vi "Update Channels on Change.vi"(10 "new channel table":T1[](array[typedef]) {"input terminal configuration" items=["default"=-1, "RSE"=10083, "NRSE"=10078, "Differential"=10106, "Pseudodifferential"=12529]; "Channel Type" items=["Voltage (V)"=0, "Charge (C)"=9, "-"=99, "SPL (Pa)"=3, "Force (lbf)"=6, "Force (N)"=1, "Acceleration (g) - IEPE"=2, "Acceleration (g) - Charge"=12, "Acceleration (g) - 4 wire DC Voltage"=22, "Velocity (in/s)"=7, "Velocity (mm/s)"=8, "Prox Probe (mil)"=4, "Prox Probe (mm)"=5]}, 11 "old channel table":T1[](array[typedef]) {"input terminal configuration" items=["default"=-1, "RSE"=10083, "NRSE"=10078, "Differential"=10106, "Pseudodifferential"=12529]; "Channel Type" items=["Voltage (V)"=0, "Charge (C)"=9, "-"=99, "SPL (Pa)"=3, "Force (lbf)"=6, "Force (N)"=1, "Acceleration (g) - IEPE"=2, "Acceleration (g) - Charge"=12, "Acceleration (g) - 4 wire DC Voltage"=22, "Velocity (in/s)"=7, "Velocity (mm/s)"=8, "Prox Probe (mil)"=4, "Prox Probe (mm)"=5]}) -> (3 "updated channel table":T1[](array[typedef]) {"input terminal configuration" items=["default"=-1, "RSE"=10083, "NRSE"=10078, "Differential"=10106, "Pseudodifferential"=12529]; "Channel Type" items=["Voltage (V)"=0, "Charge (C)"=9, "-"=99, "SPL (Pa)"=3, "Force (lbf)"=6, "Force (N)"=1, "Acceleration (g) - IEPE"=2, "Acceleration (g) - Charge"=12, "Acceleration (g) - 4 wire DC Voltage"=22, "Velocity (in/s)"=7, "Velocity (mm/s)"=8, "Prox Probe (mil)"=4, "Prox Probe (mm)"=5]})   [LabVIEW 2024, in "Dynamic Signal Acquisition (Interactive) UI.lvlib"]
uses:
  SFPDAQmx Channel Info.ctl
  <vilib>/addons/Sound and Vibration/svt_DAQmx/Configuration XControl/Controls/svx_DAQ_Excitation.ctl
  <vilib>/addons/Sound and Vibration/svt_DAQmx/Configuration XControl/Controls/svx_DAQ_Coupling.ctl
  <vilib>/addons/Sound and Vibration/svt_DAQmx/Configuration XControl/Controls/svx_DAQ_ChannelType.ctl
  <vilib>/DAQmx/create/channels.llb/DAQmx Create Channel (TEDS-AI-Sound Pressure-Microphone).vi
  <vilib>/DAQmx/create/channels.llb/DAQmx Create Channel (TEDS-AI-Force-IEPE Sensor).vi
  <vilib>/DAQmx/create/channels.llb/DAQmx Create Channel (TEDS-AI-Acceleration-Accelerometer).vi
  Dynamic Signal Acquisition (Interactive) UI.lvlib
  <vilib>/addons/Sound and Vibration/svt_DAQmx/Configuration XControl/SVX NI-DAQmx AI Configuration XControl.xctl
  <resource>/objmgr/daqmx.rc
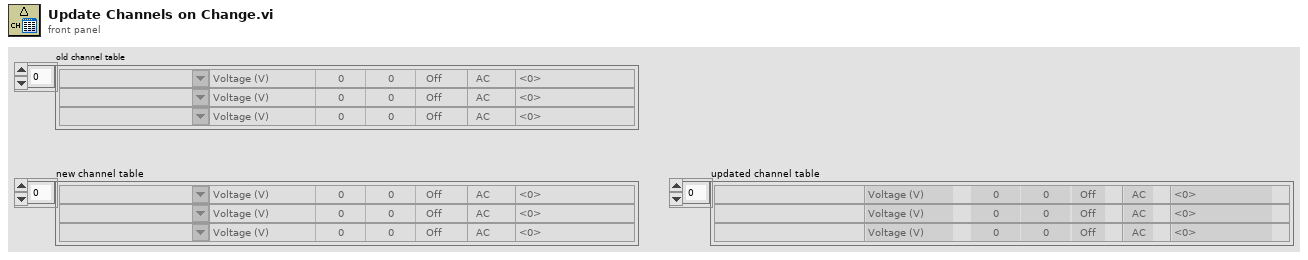
[diagram p1: front panel]
types:
  T1 = typedef "Dynamic Signal Acquisition (Interactive) UI.lvlib/SFPDAQmx Channel Info.ctl" = cluster{"DAQmx Channel":tag, "Channel Type":u16, "Max":dbl, "Sensitivity":dbl, "Coupling":enum16{"AC", "DC"}, "input terminal configuration":i32, "excitation":enum16{"Off", "Min", "Max"}}
  T2 = typedef "svx_DAQ_Excitation.ctl" = enum16{"Off", "Min", "Max"}
  T3 = typedef "SVX NI-DAQmx AI Configuration XControl.xctl/svx_DAQ_Coupling.ctl" = enum16{"AC", "DC"}
  T4 = typedef "SVX NI-DAQmx AI Configuration XControl.xctl/svx_DAQ_ChannelType.ctl" = u16
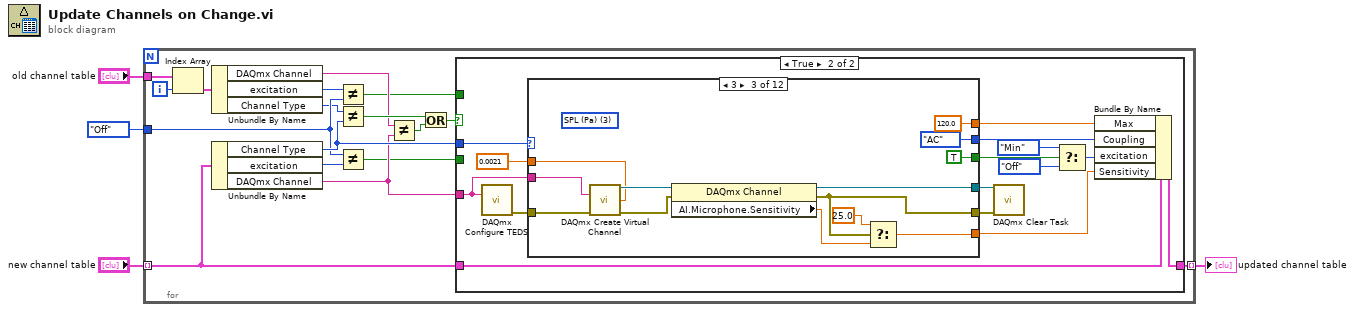
[diagram p0: block diagram]
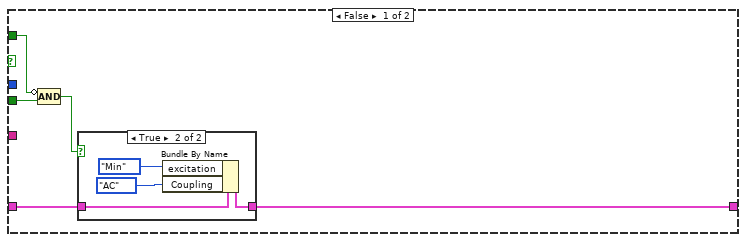
[diagram p2: hidden frame]
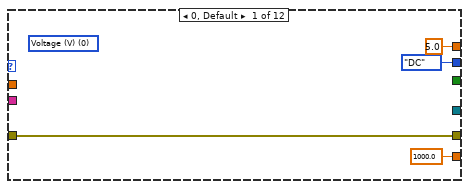
[diagram p4: hidden frame]
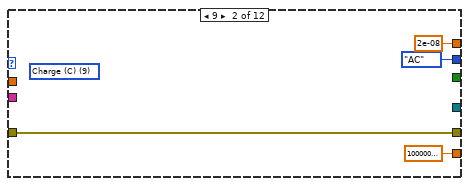
[diagram p5: hidden frame]
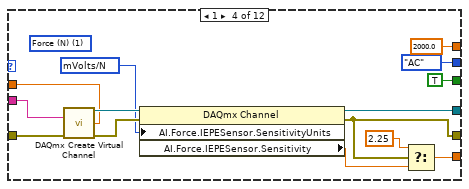
[diagram p6: hidden frame]
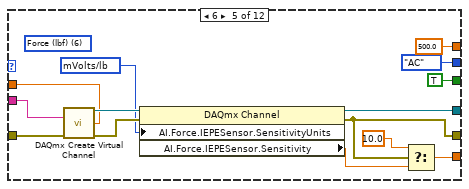
[diagram p7: hidden frame]
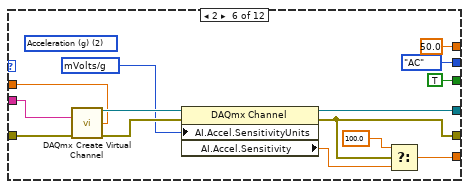
[diagram p8: hidden frame]
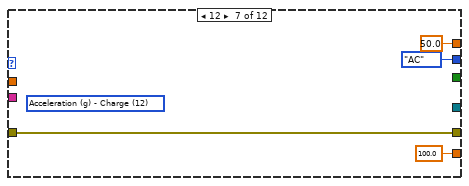
[diagram p9: hidden frame]
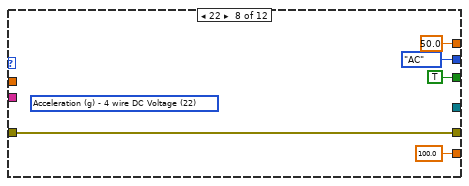
[diagram p10: hidden frame]
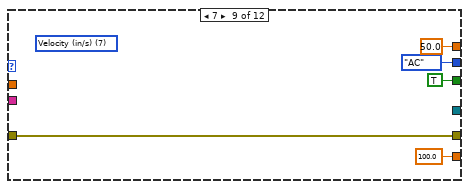
[diagram p11: hidden frame]
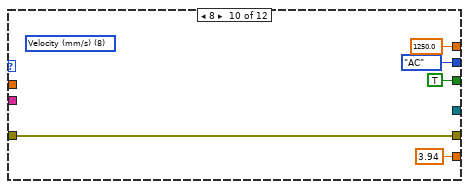
[diagram p12: hidden frame]
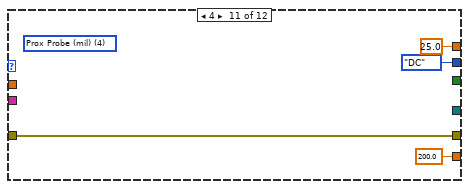
[diagram p13: hidden frame]
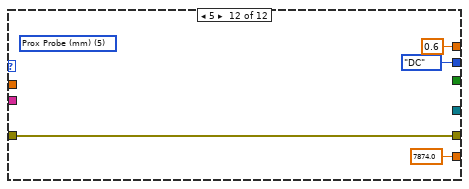
[diagram p14: hidden frame]
diagram:
  n1 = for {
    tunnel: "new channel table" -> [w21] mode=indexing
    tunnel: [w17] -> w2 mode=indexing
    tunnel: "old channel table" -> [w20]
    tunnel: svx_DAQ_Excitation."Off" ("y") -> [w13]
    i -> [w19]
    n2 = Index Array(array=w20, index=w19) -> (element=w18:T1)
    n3 = Unbundle By Name(w18) -> ("DAQmx Channel"=w10:tag, "excitation"=w14:enum16{"Off", "Min", "Max"}, "Channel Type"=w12:u16)
    n4 = Unbundle By Name(w21) -> ("Channel Type"=w16:u16, "excitation"=w15:enum16{"Off", "Min", "Max"}, "DAQmx Channel"=w9:tag)
    n5 = Not Equal?(x=w14, y=w13) -> (x != y?=w5:bool)
    n6 = Not Equal?(x=w12, y=w16) -> (x != y?=w11:bool)
    n7 = Not Equal?(x=w13, y=w15) -> (x != y?=w6:bool)
    n8 = Not Equal?(x=w10, y=w9) -> (x != y?=w8:bool)
    n9 = Or(x=w11, y=w8) -> (x .or. y?=w7:bool)
    n10 = case shown="True" w7 {
      tunnel: w21 -> [w23 w46]
      tunnel: [w22 w45] -> w17
      tunnel: w16 -> [_ w44]
      tunnel: w5 -> [w26 _]
      tunnel: w6 -> [w25 _]
      tunnel: w9 -> [_ w37]
      frame False {
        n11 = Compound Arithmetic op=AND(invert w26, w25) -> (w24:bool)
        n12 = case shown="True" w24 {
          tunnel: w23 -> [w27 w31]
          tunnel: [w27 w30] -> w22
          frame False {
          }
          frame True {
            n13 = Bundle By Name(cluster=w31, "excitation"=svx_DAQ_Excitation."Min", "Coupling"=svx_DAQ_Coupling."AC") -> (w30:T1)
          }
        }
      }
      frame True {
        n14 = call <vilib>:"DAQmx Configure TEDS.vi"("physical channel"=w37) -> ("error out"=w35:errorcluster)  [unwired: 14 in]
        n15 = case shown="3" w44 {
          tunnel: [5.0 ("Max") 2e-08 ("Max") 120.0 ("Max") 2000.0 ("Max") 500.0 ("Max") 50.0 ("Max") 50.0 ("Max") 50.0 ("Max") 50.0 ("Max") 1250.0 ("Max") 25.0 ("Max") 0.6 ("Max")] -> w43
          tunnel: [1000.0 ("Sensitivity") 1000000000000.0 ("Sensitivity") w56 w70 w83 w97 100.0 ("Sensitivity") 100.0 ("Sensitivity") 100.0 ("Sensitivity") 3.94 ("Sensitivity") 200.0 ("Sensitivity") 7874.0 ("Sensitivity")] -> w33
          tunnel: [svx_DAQ_Coupling."DC" ("Coupling") svx_DAQ_Coupling."AC" ("Coupling") svx_DAQ_Coupling."AC" ("Coupling") svx_DAQ_Coupling."AC" ("Coupling") svx_DAQ_Coupling."AC" ("Coupling") svx_DAQ_Coupling."AC" ("Coupling") svx_DAQ_Coupling."AC" ("Coupling") svx_DAQ_Coupling."AC" ("Coupling") svx_DAQ_Coupling."AC" ("Coupling") svx_DAQ_Coupling."AC" ("Coupling") svx_DAQ_Coupling."DC" ("Coupling") svx_DAQ_Coupling."DC" ("Coupling")] -> w42
          tunnel: [_ _ TRUE ("IEPE") TRUE ("IEPE") TRUE ("IEPE") TRUE ("IEPE") _ TRUE ("IEPE") TRUE ("IEPE") TRUE ("IEPE") _ _] -> w39
          tunnel: w37 -> [_ _ w64 w72 w87 w99 _ _ _ _ _ _]
          tunnel: [_ _ w62 w69 w86 w101 _ _ _ _ _ _] -> w36
          tunnel: w35 -> [w47 w51 w61 w73 w88 w102 w110 w114 w119 w124 w129 w133]
          tunnel: [w47 w51 w59 w71 w85 w100 w110 w114 w119 w124 w129 w133] -> w34
          tunnel: 0.0021 ("current excitation value") -> [_ _ w55 w68 w82 w96 _ _ _ _ _ _]
          frame 0, Default {
            (unwired) T4 0 items=["Voltage (V)"=0, "SPL (Pa)"=3, "Force (lbf)"=6, "Force (N)"=1, "Acceleration (g)"=2, "Velocity (in/s)"=7, "Velocity (mm/s)"=8, "Prox Probe (mil)"=4, "Prox Probe (mm)"=5] ("Channel Type")
          }
          frame 9 {
            (unwired) T4 9 items=["Voltage (V)"=0, "Charge (C)"=9, "-"=99, "SPL (Pa)"=3, "Force (lbf)"=6, "Force (N)"=1, "Acceleration (g) - IEPE"=2, "Acceleration (g) - Charge"=12, "Acceleration (g) - 4 wire DC Voltage"=22, "Velocity (in/s)"=7, "Velocity (mm/s)"=8, "Prox Probe (mil)"=4, "Prox Probe (mm)"=5] ("Channel Type")
          }
          frame 3 {
            (unwired) T4 3 items=["Voltage (V)"=0, "SPL (Pa)"=3, "Force (lbf)"=6, "Force (N)"=1, "Acceleration (g)"=2, "Velocity (in/s)"=7, "Velocity (mm/s)"=8, "Prox Probe (mil)"=4, "Prox Probe (mm)"=5] ("Channel Type")
            n16 = call-poly <vilib>:"DAQmx Create Virtual Channel.vi"("physical channels"=w64, "current excitation value"=w55, "error in"=w61) -> ("task out"=w63:refnum<k21>, "error out"=w60:errorcluster)  [unwired: 11 in]
            n17 = property class="DAQmx Channel"(reference=w63, error in=w60) -> (reference out=w62:refnum<k21>, error out=w59:errorcluster, "AI.Microphone.Sensitivity"=w58:dbl)
            n18 = Select(t=25.0 ("Sensitivity"), s=w59, f=w58) -> (s? t:f=w56:dbl)
          }
          frame 1 {
            w74 = 15891 items=["mVolts/N"=15891, "mVolts/lb"=15892] ("AI.Force.IEPESensor.SensitivityUnits")
            (unwired) T4 1 items=["Voltage (V)"=0, "SPL (Pa)"=3, "Force (lbf)"=6, "Force (N)"=1, "Acceleration (g)"=2, "Velocity (in/s)"=7, "Velocity (mm/s)"=8, "Prox Probe (mil)"=4, "Prox Probe (mm)"=5] ("Channel Type")
            n19 = call-poly <vilib>:"DAQmx Create Virtual Channel.vi"("physical channels"=w72, "current excitation value"=w68, "error in"=w73) -> ("task out"=w78:refnum<k21>, "error out"=w77:errorcluster)  [unwired: 11 in]
            n20 = property class="DAQmx Channel"(reference=w78, error in=w77, "AI.Force.IEPESensor.SensitivityUnits"=w74) -> (reference out=w69:refnum<k21>, error out=w71:errorcluster, "AI.Force.IEPESensor.Sensitivity"=w76:dbl)
            n21 = Select(t=2.25 ("Sensitivity"), s=w71, f=w76) -> (s? t:f=w70:dbl)
          }
          frame 6 {
            w84 = 15892 items=["mVolts/N"=15891, "mVolts/lb"=15892] ("AI.Force.IEPESensor.SensitivityUnits")
            (unwired) T4 6 items=["Voltage (V)"=0, "SPL (Pa)"=3, "Force (lbf)"=6, "Force (N)"=1, "Acceleration (g)"=2, "Velocity (in/s)"=7, "Velocity (mm/s)"=8, "Prox Probe (mil)"=4, "Prox Probe (mm)"=5] ("Channel Type")
            n22 = call-poly <vilib>:"DAQmx Create Virtual Channel.vi"("physical channels"=w87, "current excitation value"=w82, "error in"=w88) -> ("task out"=w92:refnum<k21>, "error out"=w91:errorcluster)  [unwired: 11 in]
            n23 = property class="DAQmx Channel"(reference=w92, error in=w91, "AI.Force.IEPESensor.SensitivityUnits"=w84) -> (reference out=w86:refnum<k21>, error out=w85:errorcluster, "AI.Force.IEPESensor.Sensitivity"=w90:dbl)
            n24 = Select(t=10.0 ("Sensitivity"), s=w85, f=w90) -> (s? t:f=w83:dbl)
          }
          frame 2 {
            w103 = 12509 items=["mVolts/g"=12509, "Volts/g"=12510] ("AI.Accel.SensitivityUnits")
            (unwired) T4 2 items=["Voltage (V)"=0, "SPL (Pa)"=3, "Force (lbf)"=6, "Force (N)"=1, "Acceleration (g)"=2, "Velocity (in/s)"=7, "Velocity (mm/s)"=8, "Prox Probe (mil)"=4, "Prox Probe (mm)"=5] ("Channel Type")
            n25 = call-poly <vilib>:"DAQmx Create Virtual Channel.vi"("physical channels"=w99, "current excitation value"=w96, "error in"=w102) -> ("task out"=w106:refnum<k21>, "error out"=w105:errorcluster)  [unwired: 11 in]
            n26 = property class="DAQmx Channel"(reference=w106, error in=w105, "AI.Accel.SensitivityUnits"=w103) -> (reference out=w101:refnum<k21>, error out=w100:errorcluster, "AI.Accel.Sensitivity"=w104:dbl)
            n27 = Select(t=100.0 ("Sensitivity"), s=w100, f=w104) -> (s? t:f=w97:dbl)
          }
          frame 12 {
            (unwired) T4 12 items=["Voltage (V)"=0, "Charge (C)"=9, "-"=99, "SPL (Pa)"=3, "Force (lbf)"=6, "Force (N)"=1, "Acceleration (g) - IEPE"=2, "Acceleration (g) - Charge"=12, "Acceleration (g) - 4 wire DC Voltage"=22, "Velocity (in/s)"=7, "Velocity (mm/s)"=8, "Prox Probe (mil)"=4, "Prox Probe (mm)"=5] ("Channel Type")
          }
          frame 22 {
            (unwired) T4 22 items=["Voltage (V)"=0, "Charge (C)"=9, "-"=99, "SPL (Pa)"=3, "Force (lbf)"=6, "Force (N)"=1, "Acceleration (g) - IEPE"=2, "Acceleration (g) - Charge"=12, "Acceleration (g) - 4 wire DC Voltage"=22, "Velocity (in/s)"=7, "Velocity (mm/s)"=8, "Prox Probe (mil)"=4, "Prox Probe (mm)"=5] ("Channel Type")
          }
          frame 7 {
            (unwired) T4 7 items=["Voltage (V)"=0, "SPL (Pa)"=3, "Force (lbf)"=6, "Force (N)"=1, "Acceleration (g)"=2, "Velocity (in/s)"=7, "Velocity (mm/s)"=8, "Prox Probe (mil)"=4, "Prox Probe (mm)"=5] ("Channel Type")
          }
          frame 8 {
            (unwired) T4 8 items=["Voltage (V)"=0, "SPL (Pa)"=3, "Force (lbf)"=6, "Force (N)"=1, "Acceleration (g)"=2, "Velocity (in/s)"=7, "Velocity (mm/s)"=8, "Prox Probe (mil)"=4, "Prox Probe (mm)"=5] ("Channel Type")
          }
          frame 4 {
            (unwired) T4 4 items=["Voltage (V)"=0, "SPL (Pa)"=3, "Force (lbf)"=6, "Force (N)"=1, "Acceleration (g)"=2, "Velocity (in/s)"=7, "Velocity (mm/s)"=8, "Prox Probe (mil)"=4, "Prox Probe (mm)"=5] ("Channel Type")
          }
          frame 5 {
            (unwired) T4 5 items=["Voltage (V)"=0, "SPL (Pa)"=3, "Force (lbf)"=6, "Force (N)"=1, "Acceleration (g)"=2, "Velocity (in/s)"=7, "Velocity (mm/s)"=8, "Prox Probe (mil)"=4, "Prox Probe (mm)"=5] ("Channel Type")
          }
        }
        n28 = call <vilib>:"DAQmx Clear Task.vi"("task in"=w36, "error in"=w34) -> ()  [unwired: 13 in, 1 out]
        n29 = Select(t=svx_DAQ_Excitation."Min", s=w39, f=svx_DAQ_Excitation."Off" ("excitation")) -> (s? t:f=w40:T2)
        n30 = Bundle By Name(cluster=w46, "Max"=w43, "Coupling"=w42, "excitation"=w40, "Sensitivity"=w33) -> (w45:T1)
      }
    }
  }
  "updated channel table" <- w2
